vi "Do.vi"(8 "error in (no error)":errorcluster, 10 "Actor in":refnum<class "Actor.lvclass">, 11 "DER SetpointV Msg":refnum<class "DER SetpointV Msg.lvclass">) -> (0 "error out":errorcluster, 2 "Actor out":refnum<class "Actor.lvclass">)   [LabVIEW 2018, in "EMS Core.lvlib" / "DER SetpointV Msg.lvclass"]
doc: "This VI delivers the message to the actor by calling the appropriate method(s) on the actor."
uses:
  DER SetpointV Msg.lvclass
  C:/Users/Administrator/Desktop/2018LabVIEW EMS/Device Communication and Control Abstract Actor/Device Communication and Control Abstract Messages/Set DER SetPointV Msg/Set DER SetPointV Msg.lvclass
  <vilib>/ActorFramework/Actor/Actor.lvclass
  EMS/EMS.lvclass
  C:/Program Files (x86)/National Instruments/LabVIEW 2018/vi.lib/ActorFramework/Actor/Actor.lvclass
  Device Communication and Control Abstract Actor/Device Communication and Control Abstract Messages/Set DER SetPointV Msg/Set DER SetPointV Msg.lvclass/Set DER SetPointV Msg.ctl
  Device Communication and Control Abstract Actor/Device Communication and Control Abstract Messages/Set DER SetPointV Msg/Set DER SetPointV Msg.lvclass
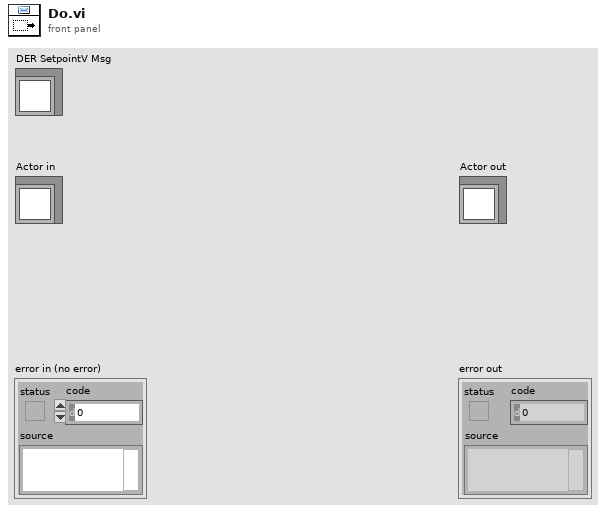
[diagram p1: front panel]
types:
  T1 = typedef "CSEISMIC DDS.lvlib/CSEISMIC DDS.lvclass/DER_SetPointV.ctl" = cluster{"DeviceID":T2, "Voltage (V)":dbl}
  T2 = typedef "CSEISMIC DDS.lvlib/CSEISMIC DDS.lvclass/DeviceID.ctl" = string
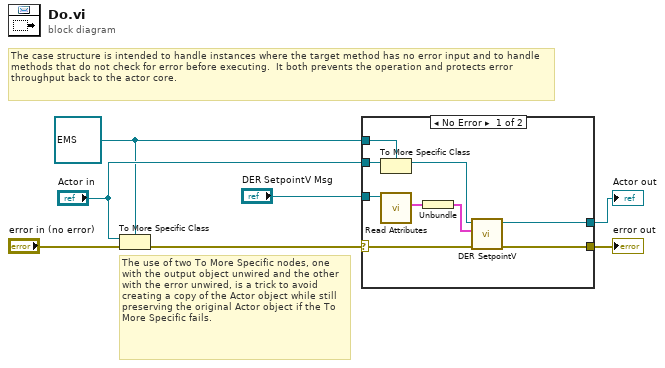
[diagram p0: block diagram]
diagram:
  w2 = refnum<class "EMS.lvclass"> refnum ("Actor in")
  # "The use of two To More Specific nodes, one with the output object unwired and the other with the error unwired, is a trick to avoid creating a copy of the Actor object while still preserving the original Actor object if the To More Specific fails."
  # "The case structure is intended to handle instances where the target method has no error input and to handle methods that do not check for error before executing.  It both prevents the operation and protects error throughput back to the actor core."
  n1 = To More Specific Class(target class=w2, reference="Actor in", error in="error in (no error)") -> (error out=w6:errorcluster)  [unwired: 1 out]
  n2 = case shown="No Error" w6 {
    selector: w6 -> [w14 w18]
    tunnel: [w16 w18] -> w5
    tunnel: [w15 w17] -> w4
    tunnel: "Actor in" -> [w13 w17]
    tunnel: w2 -> [w12 _]
    tunnel: "DER SetpointV Msg" -> [w9 _]
    frame No Error {
      n3 = To More Specific Class(target class=w12, reference=w13) -> (specific class reference=w11:refnum<class "EMS.lvclass">)  [unwired: 1 in, 1 out]
      n4 = call "Read Attributes.vi"("Set DER SetPointVF Msg"=w9) -> ("Payload"=w10:cluster{"DER_SetPointV":T1})  [unwired: 10 in]
      n5 = Unbundle(w10) -> ("DER_SetPointV"=w8:T1)
      n6 = call "DER SetpointV.vi"("error in"=w14, "DER_SetPointV"=w8, "SCADA in"=w11) -> ("error out"=w16:errorcluster, "SCADA out"=w15:refnum<class "EMS.lvclass">)  [unwired: 7 in]
    }
    frame Error {
      # "If type check fails, pass the original object out again."
    }
  }
  "error out" <- w5
  "Actor out" <- w4
